vi "List VI Hierarchy__ogtk.vi"(8 "error in (no error)":errorcluster, 9 "exclude vi.lib VIs (FALSE)":bool, 11 "VI reference":refnum<vi>) -> (0 "error out":errorcluster, 2 "Hierarchy Lists":T1, 3 "dup VI reference":refnum<vi>)   [LabVIEW 2020]
doc: "Returns a cluster of all of the Standard VIs, Control Type Definitions, Global VIs, and Polymorphic VIs in a VI's hierarchy. You may optionally exclude any VIs whose paths are in vi.lib or any of its recursive subdirectories."
panel:
  # "List VI Hierarchy.vi\n\nGets a VI's hierarchy.\n\nPlease visit http://www.OpenG.org to learn about the\nOpen Source LabVIEW software movement.\n\nNOTICE -- YOU MUST LEAVE THIS NOTICE IN PLACE.  PER THE TERMS OF THE LICENSE BELOW, YOU MAY SUBLICENSE THIS SOFTWARE \nIN ANY WAY THAT DOES NOT CONFLICT WITH THIS LICENSE.\n\n### BSD License (http://www.opensource.org/licenses/bsd-license.php) Begin ###\n \nCopyright (c) 2002, Jim Kring <jim@jimkring.com>\n\nAll rights reserved.\n\nRedistribution and use in source and binary forms, with or without modification, are permitted provided that the following conditions are met:\n\n    * Redistributions of source code must retain the above copyright notice, this list of conditions and the following disclaimer.\n    * Redistributions in binary form must reproduce the above copyright notice, this list of conditions and the following disclaimer in the \n       documentation and/or other materials provided with the distribution.\n    * Neither the name of SciWare, James Kring, Inc., nor the names of its contributors may be used to endorse or promote products derived \n       from this software without specific prior written permission.\n\nTHIS SOFTWARE IS PROVIDED BY THE COPYRIGHT HOLDERS AND CONTRIBUTORS \"AS IS\" AND ANY EXPRESS OR IMPLIED WARRANTIES, \nINCLUDING, BUT NOT LIMITED TO, THE IMPLIED WARRANTIES OF MERCHANTABILITY AND FITNESS FOR A PARTICULAR PURPOSE ARE \nDISCLAIMED. IN NO EVENT SHALL THE COPYRIGHT OWNER OR CONTRIBUTORS BE LIABLE FOR ANY DIRECT, INDIRECT, INCIDENTAL,\n SPECIAL, EXEMPLARY, OR CONSEQUENTIAL DAMAGES (INCLUDING, BUT NOT LIMITED TO, PROCUREMENT OF SUBSTITUTE GOODS OR \nSERVICES; LOSS OF USE, DATA, OR PROFITS; OR BUSINESS INTERRUPTION) HOWEVER CAUSED AND ON ANY THEORY OF LIABILITY, \nWHETHER IN CONTRACT, STRICT LIABILITY, OR TORT (INCLUDING NEGLIGENCE OR OTHERWISE) ARISING IN ANY WAY OUT OF THE USE \nOF THIS SOFTWARE, EVEN IF ADVISED OF THE POSSIBILITY OF SUCH DAMAGE.\n\n### BSD License End ###"
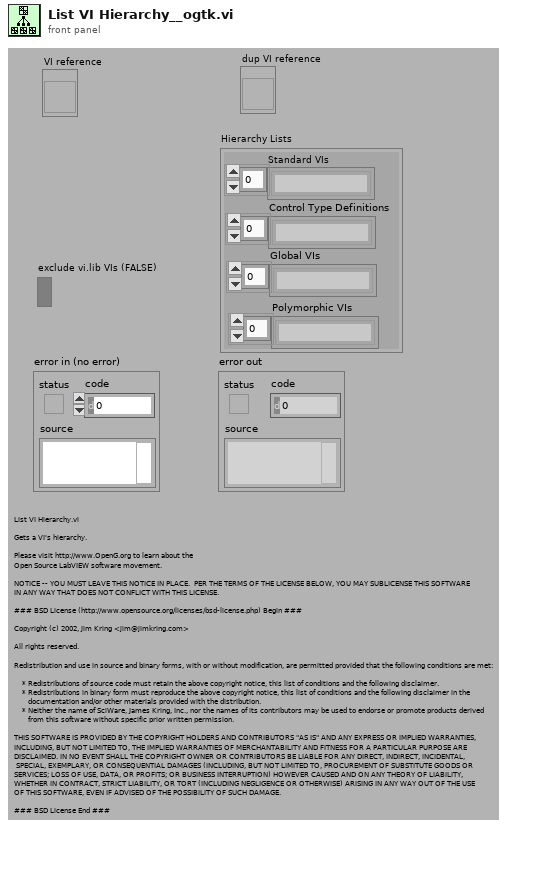
[diagram p1: front panel]
types:
  T1 = cluster{"Standard VIs":string[], "Control Type Definitions":string[], "Global VIs":string[], "Polymorphic VIs":string[]}
  T2 = enum32{"invalid VI type", "Standard VI", "Control VI", "Global VI", "Polymorphic VI", "Configuration VI", "SubSystem", "Facade VI", "Method VI", "Statechart Diagram VI"}
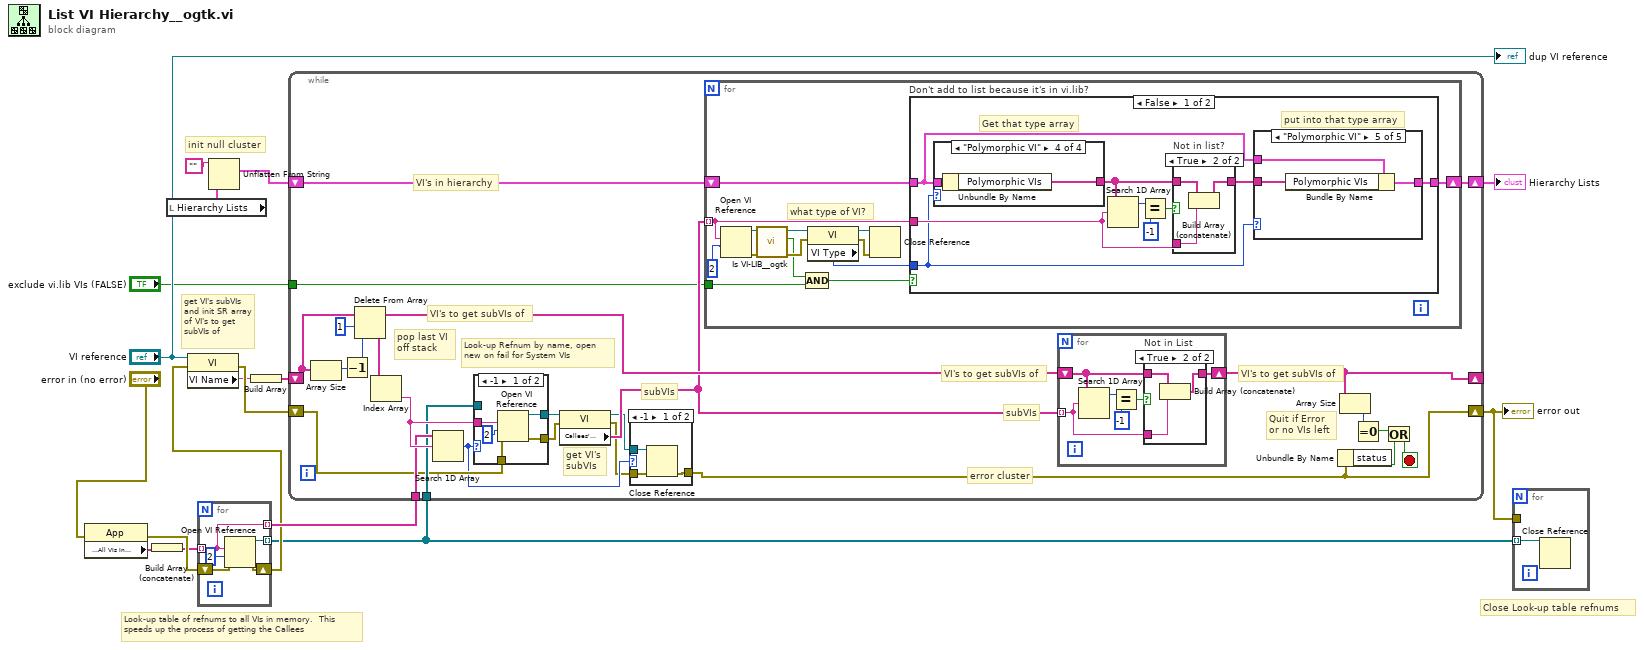
[diagram p0: block diagram]
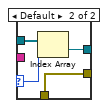
[diagram p3: hidden frame]
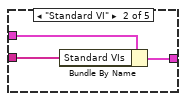
[diagram p6: hidden frame]
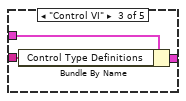
[diagram p7: hidden frame]
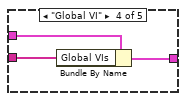
[diagram p8: hidden frame]
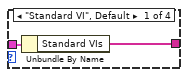
[diagram p9: hidden frame]
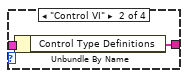
[diagram p10: hidden frame]
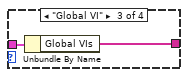
[diagram p11: hidden frame]
diagram:
  # "Close Look-up table refnums"
  # "Look-up table of refnums to all VIs in memory.  This speeds up the process of getting the Callees"
  # "get VI's subVIs and init SR array of VI's to get subVIs of"
  # "init null cluster"
  n1 = property class="App"(error in="error in (no error)") -> (error out=w8:errorcluster, "Application:All VIs In Memory"=w2:string[])  [unwired: 1 in, 1 out]
  n2 = Build Array (concatenate)(w2) -> (w1:string[])
  n3 = local read "Hierarchy Lists"() -> (w15:T1)
  n4 = for {
    tunnel: w1 -> [w19] mode=indexing
    shift-right: [w21] -> w6
    shift-left: w8 -> [w22]
    tunnel: [w20] -> w4 mode=indexing
    tunnel: [w19] -> w7 mode=indexing
    n5 = Open VI Reference(vi path=w19, options=2, error in (no error)=w22) -> (vi reference=w20:refnum<vi>, error out=w21:errorcluster)  [unwired: 3 in]
  }
  n6 = property class="VI"(reference="VI reference", error in=w6) -> (error out=w17:errorcluster, "VI Name"=w10:string)  [unwired: 1 out]
  n7 = Unflatten From String(type=w15, binary string="") -> (value=w13:T1)  [unwired: 3 in, 2 out]
  n8 = Build Array(w10) -> (w9:string[])
  n9 = while {
    tunnel: w4 -> [w30]
    tunnel: w7 -> [w31]
    tunnel: "exclude vi.lib VIs (FALSE)" -> [w33]
    shift-left: w17 -> [w28]
    shift-right: [w23] -> w3
    shift-left: w13 -> [w38]
    shift-right: [w37] -> w12
    shift-left: w9 -> [w39]
    shift-right: [w35] -> _
    stop <- w42 stop-if-true
    # "Look-up Refnum by name, open new on fail for System VIs"
    # "error cluster"
    # "VI's to get subVIs of"
    # "subVIs"
    # "subVIs"
    # "VI's to get subVIs of"
    # "VI's to get subVIs of"
    # "get VI's subVIs"
    # "pop last VI off stack"
    # "Quit if Error or no VIs left"
    # "VI's in hierarchy"
    n10 = Array Size(array=w39) -> (size(s)=w40:i32)
    n11 = Decrement(x=w40) -> (x-1=w41:i32)
    n12 = Delete From Array(array=w39, length=1 ("Length"), index=w41) -> (deleted portion=w46:string[], array with subset deleted=w36:string[])
    n13 = Index Array(array=w46) -> (element=w32:string)  [unwired: 1 in]
    n14 = Search 1D Array(1D array=w31, element=w32) -> (index of element=w25:i32)  [unwired: 1 in]
    n15 = case shown="-1" w25 {
      selector: w25 -> [_ w58]
      tunnel: w30 -> [_ w60]
      tunnel: [w56 w59] -> w29
      tunnel: w32 -> [w55 _]
      tunnel: [w54 w57] -> w27
      tunnel: w28 -> [w53 w57]
      frame -1 {
        n16 = Open VI Reference(vi path=w55, options=2, error in (no error)=w53) -> (vi reference=w56:refnum<vi>, error out=w54:errorcluster)  [unwired: 3 in]
      }
      frame Default {
        n17 = Index Array(array=w60, index=w58) -> (element=w59:refnum<vi>)
      }
    }
    n18 = property class="VI"(reference=w29, error in=w27) -> (reference out=w26:refnum<vi>, error out=w24:errorcluster, "Callees' Names"=w34:string[])
    n19 = case shown="-1" w25 {
      tunnel: w26 -> [w50 _]
      tunnel: [w49 w51] -> w23
      tunnel: w24 -> [w48 w51]
      frame -1 {
        n20 = Close Reference(reference=w50, error in (no error)=w48) -> (error out=w49:errorcluster)
      }
      frame Default {
      }
    }
    n21 = for {
      tunnel: w34 -> [w82] mode=indexing
      shift-right: [w79] -> w37
      shift-left: w38 -> [w80]
      tunnel: w33 -> [w73]
      # "what type of VI?"
      n22 = Open VI Reference(vi path=w82, options=2) -> (vi reference=w78:refnum<vi>, error out=w75:errorcluster)  [unwired: 4 in]
      n23 = call <userlib>:"Is VI-LIB__ogtk.vi"("error in (no error)"=w75, "VI reference"=w78) -> ("error out"=w76:errorcluster, "is vi.lib?"=w74:bool, "dup VI reference"=w77:refnum<vi>)  [unwired: 7 in]
      n24 = Compound Arithmetic op=AND(w74, w73) -> (w72:bool)
      n25 = property class="VI"(reference=w77, error in=w76) -> (reference out=w84:refnum<vi>, error out=w83:errorcluster, "VI Type"=w81:T2)
      n26 = Close Reference(reference=w84, error in (no error)=w83) -> ()  [unwired: 1 out]
      n27 = case "Don't add to list because it's in vi.lib?" shown="False" w72 {
        tunnel: w82 -> [w90 _]
        tunnel: w81 -> [w88 _]
        tunnel: w80 -> [w87 w119]
        tunnel: [w86 w119] -> w79
        frame False {
          # "put into that type array"
          # "Get that type array"
          n28 = case shown="\"Polymorphic VI\"" w88 {
            tunnel: w87 -> [w108 w110 w112 w114]
            tunnel: [w107 w109 w111 w113] -> w89
            frame "Standard VI", Default {
              n29 = Unbundle By Name(w108) -> ("Standard VIs"=w107:string[])
            }
            frame "Control VI" {
              n30 = Unbundle By Name(w110) -> ("Control Type Definitions"=w109:string[])
            }
            frame "Global VI" {
              n31 = Unbundle By Name(w112) -> ("Global VIs"=w111:string[])
            }
            frame "Polymorphic VI" {
              n32 = Unbundle By Name(w114) -> ("Polymorphic VIs"=w113:string[])
            }
          }
          n33 = Search 1D Array(1D array=w89, element=w90) -> (index of element=w93:i32)  [unwired: 1 in]
          n34 = Equal?(x=w93, y=-1) -> (x = y?=w91:bool)
          n35 = case "Not in list?" shown="True" w91 {
            tunnel: w89 -> [w115 w118]
            tunnel: w90 -> [_ w117]
            tunnel: [w115 w116] -> w85
            frame False {
            }
            frame True {
              n36 = Build Array (concatenate)(w118, w117) -> (w116:string[])
            }
          }
          n37 = case shown="\"Polymorphic VI\"" w88 {
            tunnel: w87 -> [w94 w97 w100 w103 w106]
            tunnel: [w94 w95 w98 w101 w104] -> w86
            tunnel: w85 -> [_ w96 w99 w102 w105]
            frame Default {
            }
            frame "Standard VI" {
              n38 = Bundle By Name(cluster=w97, "Standard VIs"=w96) -> (w95:T1)
            }
            frame "Control VI" {
              n39 = Bundle By Name(cluster=w100, "Control Type Definitions"=w99) -> (w98:T1)
            }
            frame "Global VI" {
              n40 = Bundle By Name(cluster=w103, "Global VIs"=w102) -> (w101:T1)
            }
            frame "Polymorphic VI" {
              n41 = Bundle By Name(cluster=w106, "Polymorphic VIs"=w105) -> (w104:T1)
            }
          }
        }
        frame True {
        }
      }
    }
    n42 = for {
      tunnel: w34 -> [w62] mode=indexing
      shift-right: [w61] -> w35
      shift-left: w36 -> [w63]
      n43 = Search 1D Array(1D array=w63, element=w62) -> (index of element=w66:i32)  [unwired: 1 in]
      n44 = Equal?(x=w66, y=-1) -> (x = y?=w64:bool)
      n45 = case "Not in List" shown="True" w64 {
        tunnel: w63 -> [w67 w70]
        tunnel: w62 -> [_ w69]
        tunnel: [w67 w68] -> w61
        frame False {
        }
        frame True {
          n46 = Build Array (concatenate)(w70, w69) -> (w68:string[])
        }
      }
    }
    n47 = Unbundle By Name(w23) -> ("status"=w44:bool)
    n48 = Array Size(array=w35) -> (size(s)=w45:i32)
    n49 = Equal To 0?(x=w45) -> (x = 0?=w43:bool)
    n50 = Or(x=w43, y=w44) -> (x .or. y?=w42:bool)
  }
  "error out" <- w3
  "Hierarchy Lists" <- w12
  n51 = for {
    tunnel: w4 -> [w120] mode=indexing
    tunnel: w3 -> [_]
    n52 = Close Reference(reference=w120) -> ()  [unwired: 1 in, 1 out]
  }
  "dup VI reference" <- "VI reference"
